vi "EventInfoVIRunning.vi"(8 "error in (no error)":errorcluster, 10 "OnOff":bool, 11 "name":string="name") -> (0 "error out":errorcluster, 3 "eventinfoJSON":variant)   [LabVIEW 2018]
uses:
  <vilib>/LVH/i3 JSON/JSON Generation/Create Value Files/Create Value - Object.vi
  <vilib>/LVH/i3 JSON/JSON Generation/Add Object Parameter Files/Add Object Parameter - String.vi
  <vilib>/LVH/i3 JSON/JSON Generation/Add Object Parameter Files/Add Object Parameter - Boolean.vi
  <vilib>/LVH/i3 JSON/JSON Generation/Add Object Parameter Files/Add Object Parameter - Object.vi
  <vilib>/LVH/i3 JSON/i3-json.lvlib
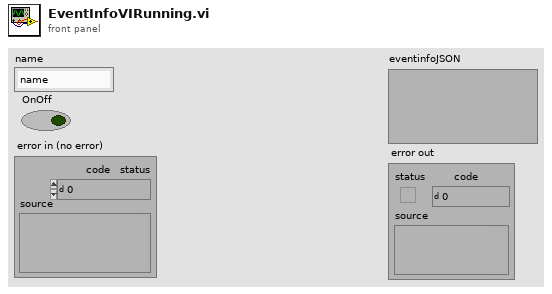
[diagram p1: front panel]
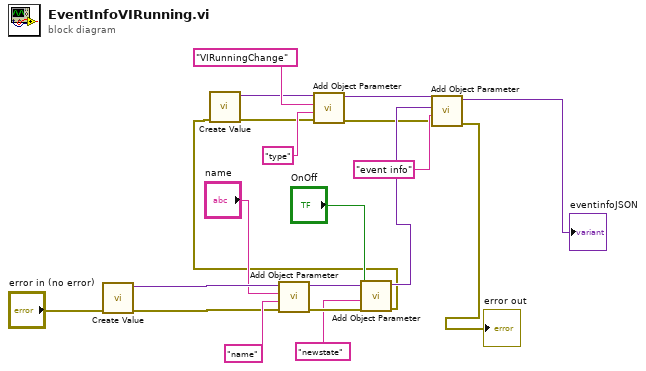
[diagram p0: block diagram]
diagram:
  n1 = call-poly <vilib>:"Create Value.vi"("error in (no error)"="error in (no error)") -> ("error out"=w17:errorcluster, "JSON Tree"=w20:variant)  [unwired: 9 in]
  n2 = call-poly <vilib>:"Add Object Parameter.vi"("error in (no error)"=w17, "Name"="name", "String"="name", "JSON Tree in (JSON Object)"=w20) -> ("error out"=w15:errorcluster, "JSON Tree out (JSON Object)"=w16:variant)  [unwired: 6 in]
  n3 = call-poly <vilib>:"Add Object Parameter.vi"("error in (no error)"=w15, "Name"="newstate", "Boolean"="OnOff", "JSON Tree in (JSON Object)"=w16) -> ("error out"=w2:errorcluster, "JSON Tree out (JSON Object)"=w11:variant)  [unwired: 6 in]
  n4 = call-poly <vilib>:"Create Value.vi"("error in (no error)"=w2) -> ("error out"=w6:errorcluster, "JSON Tree"=w7:variant)  [unwired: 9 in]
  n5 = call-poly <vilib>:"Add Object Parameter.vi"("error in (no error)"=w6, "Name"="type", "String"="VIRunningChange", "JSON Tree in (JSON Object)"=w7) -> ("error out"=w4:errorcluster, "JSON Tree out (JSON Object)"=w5:variant)  [unwired: 6 in]
  n6 = call-poly <vilib>:"Add Object Parameter.vi"("error in (no error)"=w4, "Name"="event info", "JSON Object"=w11, "JSON Tree in (JSON Object)"=w5) -> ("error out"=→"error out":errorcluster, "JSON Tree out (JSON Object)"=→"eventinfoJSON":variant)  [unwired: 6 in]
